vi "Heater Control.vi"(2 "error in (no error)":errorcluster, 3 "Heater Level":enum16{"Off", "Medium", "Maximum"}(ring), 4 "Physical Channel Read":tag, 5 "Physical Channel Write":tag) -> (0 "error out":errorcluster, 1 "Heater Level (V)":dbl format="%#.3f")   [LabVIEW 2021]
doc: "Controla la temperatura del calentador de una DAQ a partir del nivel deseado pasado por Heater Level"
uses:
  <vilib>/DAQmx/write.llb/DAQmx Write (Analog DBL 1Chan 1Samp).vi
  <vilib>/DAQmx/read.llb/DAQmx Read (Analog 1D DBL 1Chan NSamp).vi
  <vilib>/Analysis/baseanly.llb/Mean (DBL).vi
  <vilib>/DAQmx/create/channels.llb/DAQmx Create Channel (AO-Voltage-Basic).vi
  <vilib>/DAQmx/miscellaneous.llb/DAQmx Fill In Error Info.vi
  <vilib>/DAQmx/create/channels.llb/DAQmx Create Channel (AI-Voltage-Basic).vi
  <vilib>/DAQmx/configure/timing.llb/DAQmx Timing (Sample Clock).vi
  <vilib>/Analysis/NI_AALBase.lvlib
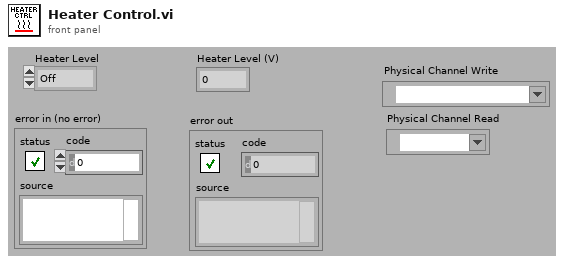
[diagram p1: front panel]
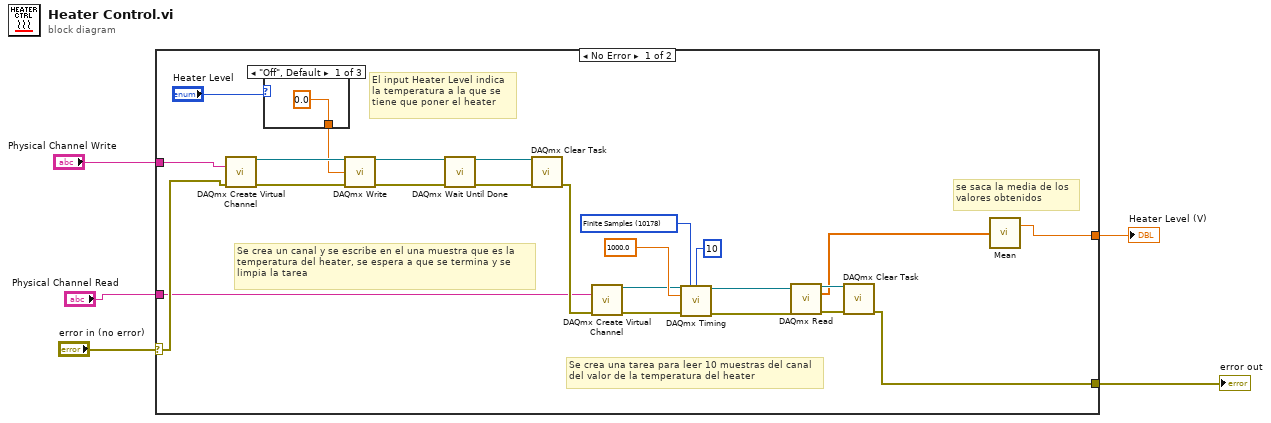
[diagram p0: block diagram]
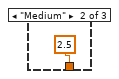
[diagram p2: hidden frame]
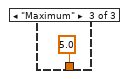
[diagram p3: hidden frame]
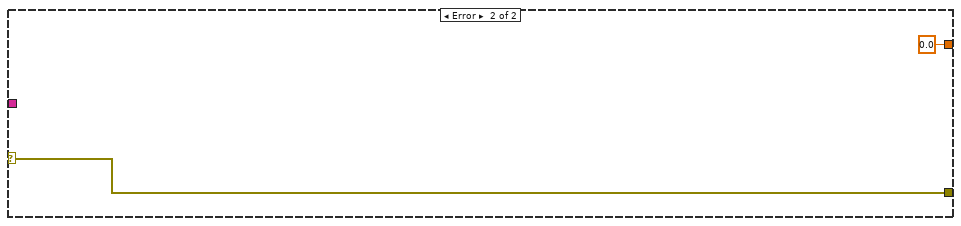
[diagram p4: hidden frame]
diagram:
  n1 = case shown="No Error" "error in (no error)" {
    selector: "error in (no error)" -> [w29 w34]
    tunnel: [w18 w34] -> w4
    tunnel: [w7 0.0 ("data")] -> w3
    tunnel: "Physical Channel Read" -> [w19 _]
    tunnel: "Physical Channel Write" -> [w15 _]
    frame No Error {
      w11 = 10178 items=["Finite Samples"=10178, "Continuous Samples"=10123, "Hardware Timed Single Point"=12522] ("sample mode")
      # "se saca la media de los \nvalores obtenidos"
      # "Se crea una tarea para leer 10 muestras del canal\ndel valor de la temperatura del heater"
      # "Se crea un canal y se escribe en el una muestra que es la \ntemperatura del heater, se espera a que se termina y se \nlimpia la tarea"
      # "El input Heater Level indica\nla temperatura a la que se \ntiene que poner el heater"
      n2 = call-poly <vilib>:"DAQmx Create Virtual Channel.vi"("physical channels"=w15, "error in"=w29) -> ("task out"=w25:refnum<k21>, "error out"=w28:errorcluster)  [unwired: 12 in]
      n3 = case shown="\"Off\", Default" "Heater Level" {
        tunnel: [0.0 2.5 5.0] -> w16
        frame "Off", Default {
        }
        frame "Medium" {
        }
        frame "Maximum" {
        }
      }
      n4 = call-poly <vilib>:"DAQmx Write.vi"("task/channels in"=w25, "data"=w16, "error in"=w28) -> ("task out"=w24:refnum<k21>, "error out"=w27:errorcluster)  [unwired: 10 in, 1 out]
      n5 = call <vilib>:"DAQmx Wait Until Done.vi"("task/channels in"=w24, "error in"=w27) -> ("task out"=w23:refnum<k21>, "error out"=w26:errorcluster)  [unwired: 12 in]
      n6 = call <vilib>:"DAQmx Clear Task.vi"("task in"=w23, "error in"=w26) -> ("error out"=w22:errorcluster)  [unwired: 13 in]
      n7 = call-poly <vilib>:"DAQmx Create Virtual Channel.vi"("physical channels"=w19, "error in"=w22) -> ("task out"=w13:refnum<k21>, "error out"=w12:errorcluster)  [unwired: 12 in]
      n8 = call-poly <vilib>:"DAQmx Timing.vi"("task/channels in"=w13, "sample mode"=w11, "samples per channel"=10, "rate"=1000.0, "error in"=w12) -> ("task out"=w9:refnum<k21>, "error out"=w8:errorcluster)  [unwired: 9 in]
      n9 = call-poly <vilib>:"DAQmx Read.vi"("task/channels in"=w9, "error in"=w8) -> ("task out"=w20:refnum<k21>, "data"=w6:dbl[], "error out"=w21:errorcluster)  [unwired: 11 in]
      n10 = call <vilib>:"DAQmx Clear Task.vi"("task in"=w20, "error in"=w21) -> ("error out"=w18:errorcluster)  [unwired: 13 in]
      n11 = call-poly <vilib>:"Mean.vi"("X"=w6) -> ("mean"=w7:dbl)  [unwired: 1 out]
    }
    frame Error {
    }
  }
  "error out" <- w4
  "Heater Level (V)" <- w3
